vi "Set_API_Mode.vi"(2 "Wait for Input":bool, 3 "API Blocking":bool, 4 "API Mode":T1(ring), 5 "Argument List In":string[](array[string])) -> (1 "Argument List Out":string[](array[string]))   [LabVIEW 2011]
doc: "This VI sets the API mode via an argument list. There are three API modes: Discrete, Continuous, and Instantaneous. Discrete mode uses two discrete start/end commands which call their respective states, with the run state executing with the main loop. Continuous mode Uses only one command to execute the start state, then runs continuously with the main loop until another command of the same class is encountered or the sequence terminates. Instantaneous mode only executes the start state once."
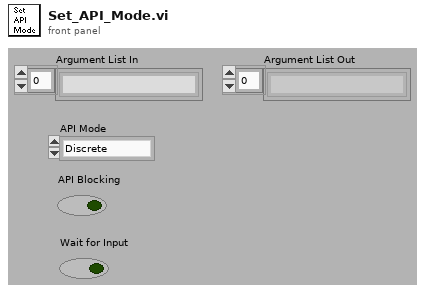
[diagram p1: front panel]
types:
  T1 = enum16{"Discrete", "Continuous", "Instantaneous", "Finite"}
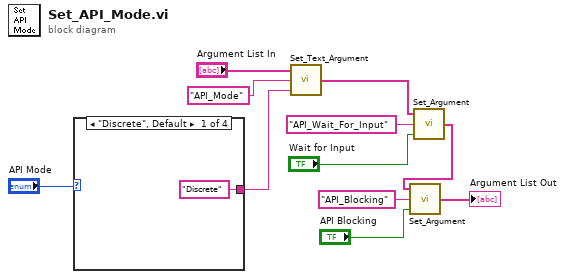
[diagram p0: block diagram]
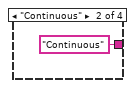
[diagram p2: hidden frame]
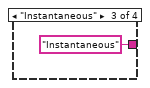
[diagram p3: hidden frame]
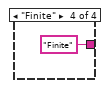
[diagram p4: hidden frame]
diagram:
  n1 = case shown="\"Discrete\", Default" "API Mode" {
    tunnel: ["Discrete" ("String") "Continuous" ("String") "Instantaneous" ("String") "Finite" ("String")] -> w8
    frame "Discrete", Default {
    }
    frame "Continuous" {
    }
    frame "Instantaneous" {
    }
    frame "Finite" {
    }
  }
  n2 = call "Set_Text_Argument.vi"("Text"=w8, "Argument"="API_Mode", "Argument List In"="Argument List In") -> ("Argument List Out"=w7:string[])
  n3 = call "Set_Argument.vi"("Enable"="Wait for Input", "Argument"="API_Wait_For_Input", "Argument List In"=w7) -> ("Argument List Out"=w4:string[])
  n4 = call "Set_Argument.vi"("Enable"="API Blocking", "Argument"="API_Blocking", "Argument List In"=w4) -> ("Argument List Out"=→"Argument List Out":string[])
